vi "获取启动参数.vi"(7 "MB通信方式选择":enum16{"串口", "TCP"}(ring), 8 "Error in":errorcluster caption="Error in (no error)", 9 "Port (502)":u16=502, 10 "IP Address":string="localhost", 11 "VISA Resource":refnum<visa-resource-name>) -> (0 "error out":errorcluster, 3 "数组":cluster{"String":string, "Value":u16}[](array[cluster]))   [LabVIEW 2016, in "斯坦道通用流路CODmn.lvlib"]
uses:
  <vilib>/Plasmionique/MB Master/MB_Master_Serial/MB_Master_Serial.lvclass
  E:/Program Files (x86)/National Instruments/LabVIEW 2016/vi.lib/Plasmionique/MB Master/MB_Master/MB_Master.lvclass
  <vilib>/Plasmionique/MB Master/MB_Master_TCP/MB_Master_TCP.lvclass
  <vilib>/Plasmionique/MB Master/MB_Master/MB_Master.lvclass
  <vilib>/Plasmionique/MB Master/MB Master.lvlib
panel:
  out "为空？":bool
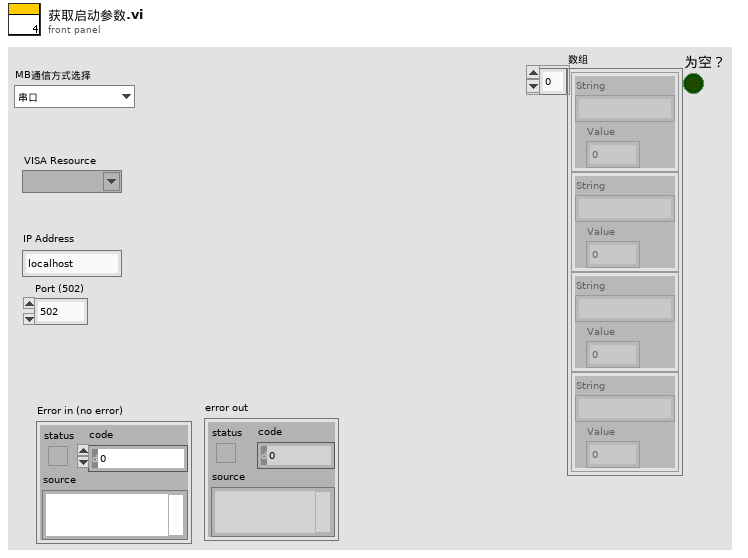
[diagram p1: front panel]
types:
  T1 = cluster{"baud rate (bps)":u32, "stop bits":u16, "parity":u16, "flow control":u16, "timeout":u32, "retries":i32}
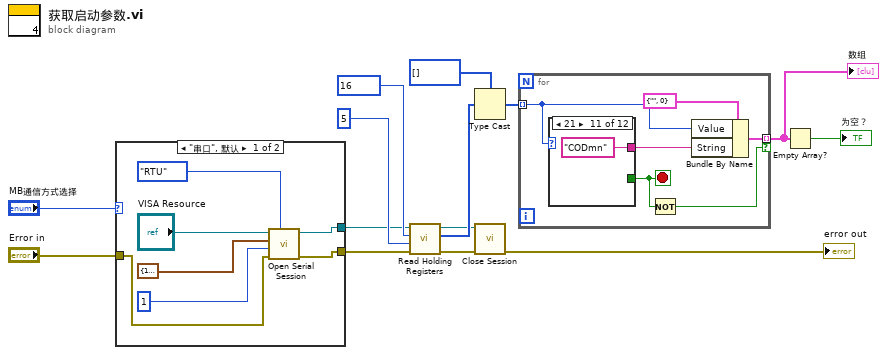
[diagram p0: block diagram]
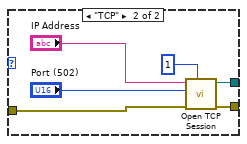
[diagram p2: hidden frame]
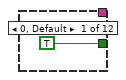
[diagram p3: hidden frame]
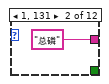
[diagram p4: hidden frame]
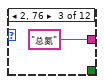
[diagram p5: hidden frame]
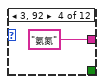
[diagram p6: hidden frame]
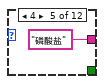
[diagram p7: hidden frame]
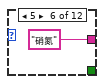
[diagram p8: hidden frame]
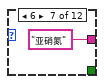
[diagram p9: hidden frame]
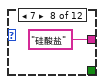
[diagram p10: hidden frame]
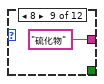
[diagram p11: hidden frame]
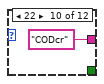
[diagram p12: hidden frame]
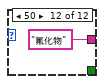
[diagram p13: hidden frame]
diagram:
  n1 = case shown="\"串口\", 默认" "MB通信方式选择" {
    tunnel: [w21 w27] -> w9
    tunnel: "Error in" -> [w16 w25]
    tunnel: [w15 w26] -> w6
    frame "串口", Default {
      n2 = call <vilib>:"Open Serial Session.vi"("Mode (RTU)"=enum16{"RTU", "ASCII"}."RTU", "Error in"=w16, "Slave ID"=u8 1, "Serial Config"=T1 {"baud rate (bps)"=115200, "stop bits"=10, "parity"=0, "flow control"=0, "timeout"=1000, "retries"=1}, "VISA Resource"="VISA Resource") -> ("Error out"=w15:errorcluster, "MB_Serial session"=w21:refnum<class "MB_Master_Serial.lvclass">)  [unwired: 5 in]
    }
    frame "TCP" {
      n3 = call <vilib>:"Open TCP Session.vi"("Slave ID (255)"=u8 1, "error in (no error)"=w25, "Port (502)"="Port (502)", "IP Address"="IP Address") -> ("error out"=w26:errorcluster, "MB_TCP session"=w27:refnum<class "MB_Master_TCP.lvclass">)  [unwired: 6 in]
    }
  }
  n4 = call <vilib>:"Read Holding Registers.vi"("error in (no error)"=w6, "quantity"=u16 5, "starting address"=u16 16, "MB session in"=w9) -> ("error out"=w5:errorcluster, "Registers"=w12:u16[], "MB session out"=w8:refnum<class "MB_Master.lvclass">)  [unwired: 5 in]
  n5 = Type Cast(type=u8[] [], x=w12) -> (*(type *) &x=w10:u8[])
  n6 = call-dynamic "Close Session.vi"("error in (no error)"=w5, "MB session in"=w8) -> ("error out"=→"error out":errorcluster)  [unwired: 9 in]
  n7 = for {
    tunnel: w10 -> [w30] mode=indexing
    tunnel: [w29] -> w2 mode=indexing if=w28
    stop <- w33 stop-if-true
    n8 = case shown="21" w30 {
      tunnel: [_ "总磷" ("table输入") "总氮" ("table输入") "氨氮" ("table输入") "磷酸盐" ("table输入") "硝氮" ("table输入") "亚硝氮" ("table输入") "硅酸盐" ("table输入") "硫化物" ("table输入") "CODcr" ("table输入") "CODmn" ("table输入") "氟化物" ("table输入")] -> w31
      tunnel: [TRUE _ _ _ _ _ _ _ _ _ _ _] -> w33
      frame 0, Default {
      }
      frame 1, 131 {
      }
      frame 2, 76 {
      }
      frame 3, 92 {
      }
      frame 4 {
      }
      frame 5 {
      }
      frame 6 {
      }
      frame 7 {
      }
      frame 8 {
      }
      frame 22 {
      }
      frame 21 {
      }
      frame 50 {
      }
    }
    n9 = Not(x=w33) -> (.not. x?=w28:bool)
    n10 = Bundle By Name(cluster=cluster{"String":string, "Value":u16} {"String"="", "Value"=0}, "Value"=w30, "String"=w31) -> (w29:cluster{"String":string, "Value":u16})
  }
  "数组" <- w2
  n11 = Empty Array?(array=w2) -> (empty?=→"为空？":bool)
